vi "Cryo-Con Set Loop Type.vi"(8 "error in (no error)":errorcluster, 10 "Set T":T1=enum."Manual", 11 "VISA Resource Name":refnum<visa-resource-name>) -> (0 "error out":errorcluster, 3 "VISA Resource Name Out":refnum<visa-resource-name>)   [LabVIEW 2015]
uses:
  Cry-Con Loop Type.ctl
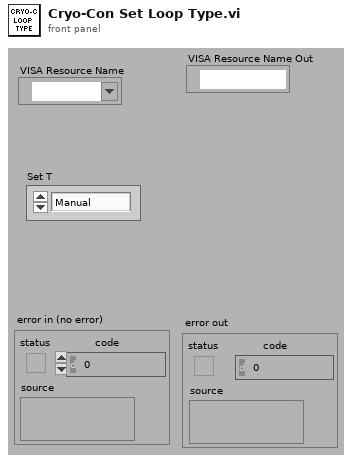
[diagram p1: front panel]
types:
  T1 = typedef "Cry-Con Loop Type.ctl" = enum16{"Off", "PID", "Manual", "PID Table", "PID Ramp", "PID Table Ramp"}
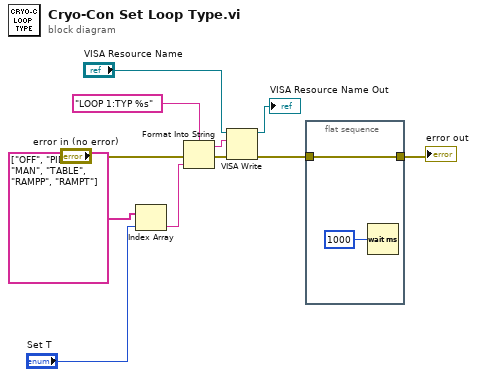
[diagram p0: block diagram]
diagram:
  n1 = Index Array(array=string[] ["OFF", "PID", "MAN", "TABLE", "RAMPP", "RAMPT"] ("string array"), index="Set T") -> (element=w4:string)
  n2 = Format Into String(format string="LOOP 1:TYP %s", error in="error in (no error)", w4) -> (resulting string=w8:string, error out=w10:errorcluster)  [unwired: 1 in]
  n3 = VISA Write(VISA resource name="VISA Resource Name", write buffer=w8, error in (no error)=w10) -> (VISA resource name out=→"VISA Resource Name Out":refnum<visa-resource-name>, error out=w2:errorcluster)  [unwired: 1 out]
  n4 = flat-sequence {
    tunnel: w2 -> [w13]
    tunnel: [w13] -> w1
    frame #0 {
      n5 = Wait (ms)(milliseconds to wait=u32 1000) -> ()  [unwired: 1 out]
    }
  }
  "error out" <- w1
